vi "Digital Write Multiple Channels.vi"(8 "error in (no error)":errorcluster, 9 "Values":bool[](array[boolean]), 10 "Indices":i32[](array[numeric]), 11 "NI-DAQ in":refnum<class "NI-DAQ.lvclass">) -> (0 "error out":errorcluster, 3 "NI-DAQ out":refnum<class "NI-DAQ.lvclass">)   [LabVIEW 2021, in "NI-DAQ.lvclass"]
uses:
  NI-DAQ.lvclass
  NI-DAQ.lvclass/NI-DAQ.ctl
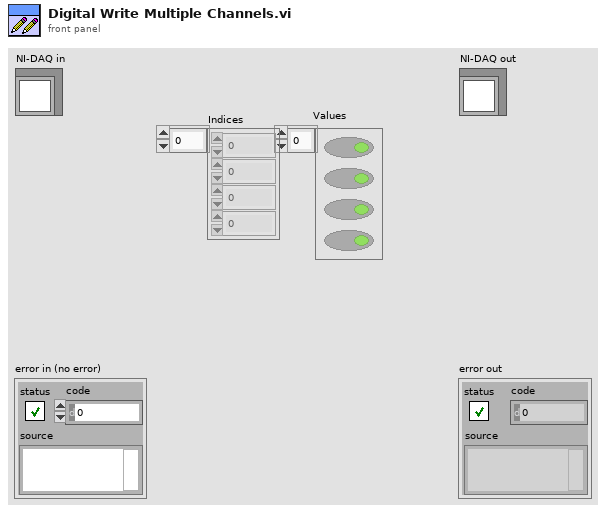
[diagram p1: front panel]
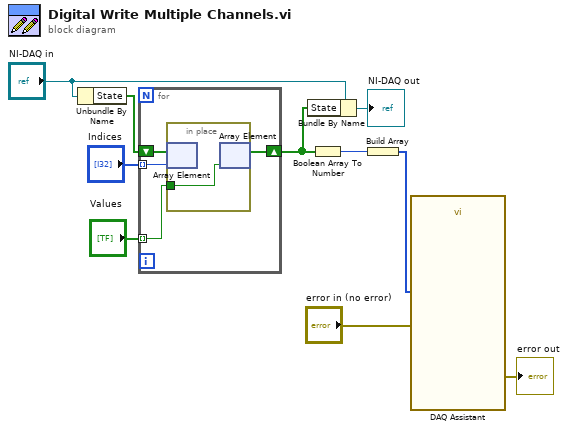
[diagram p0: block diagram]
diagram:
  n1 = Unbundle By Name("NI-DAQ in") -> ("State"=w4:bool[])
  n2 = for {
    tunnel: "Values" -> [w14] mode=indexing
    tunnel: "Indices" -> [w13] mode=indexing
    shift-right: [w11] -> w3
    shift-left: w4 -> [w12]
    n3 = in-place {
      in-place-border: w14 -> [w15]
      n4 = in-place-array #1(w12, w13) -> ()  [unwired: 1 out]
      n5 = in-place-array #1(w15) -> (w11:bool[])  [unwired: 1 out]
    }
  }
  n6 = Bundle By Name(cluster="NI-DAQ in", "State"=w3) -> (→"NI-DAQ out":refnum<class "NI-DAQ.lvclass">)
  n7 = Boolean Array To Number(Boolean array=w3) -> (number=w10:u32)
  n8 = Build Array(w10) -> (w9:u32[])
  n9 = call "DAQ Assistant"("data"=w9, "error in"="error in (no error)") -> ("error out"=→"error out":errorcluster)  [unwired: 16 in, 1 out]
